vi "Update Application Settings.vi"(6 "wait for reply (T)":bool=TRUE, 8 "error in":errorcluster) -> (0 "error out":errorcluster, 1 "timed out?":bool, 2 "Reply Payload":T1)   [LabVIEW 2020, in "Settings Editor.lvlib"]
doc: "Request Settings Editor to return the latest settings. The Settings Editor can send the applications settings as a reply or via broadcast.\n_____\nCreated using DQMH Event Scripter 4.1.0.75.\n_____\nBased on DQMH Project Template 7.0.1.1316."
uses:
  Settings Editor.lvlib
  Update Application Settings (Reply Payload)--cluster.ctl
  Settings--cluster.ctl
  CML Shared/Signal Type--enum.ctl
  CML Shared/Calibration Values--cluster.ctl
  Update Application Settings Argument--cluster.ctl
  CML Shared/CML Shared.lvlib
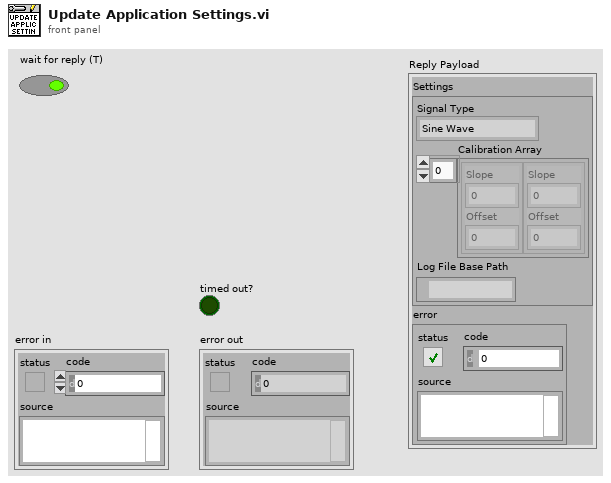
[diagram p1: front panel]
types:
  T1 = typedef "Settings Editor.lvlib/Update Application Settings (Reply Payload)--cluster.ctl" = cluster{"Settings":T2, "error":errorcluster}
  T2 = typedef "Settings Editor.lvlib/Settings--cluster.ctl" = cluster{"Signal Type":T3, "Calibration Array":T4[], "Log File Base Path":path}
  T3 = typedef "CML Shared.lvlib/Signal Type--enum.ctl" = enum16{"Sine Wave", "Square with Noise"}
  T4 = typedef "CML Shared.lvlib/Calibration Values--cluster.ctl" = cluster{"Slope":dbl, "Offset":dbl}
  T5 = typedef "Settings Editor.lvlib/Request Events--cluster.ctl" = cluster{"Stop Module":refnum<user-event>, "Show Panel":refnum<user-event>, "Hide Panel":refnum<user-event>, "Get Module Execution Status":refnum<user-event>, "Show Diagram":refnum<user-event>, "Update Application Settings":refnum<user-event>}
  T6 = typedef "Settings Editor.lvlib/Update Application Settings Argument--cluster.ctl" = cluster{"Wait Notifier":refnum<notifier>, "wait for reply":bool}
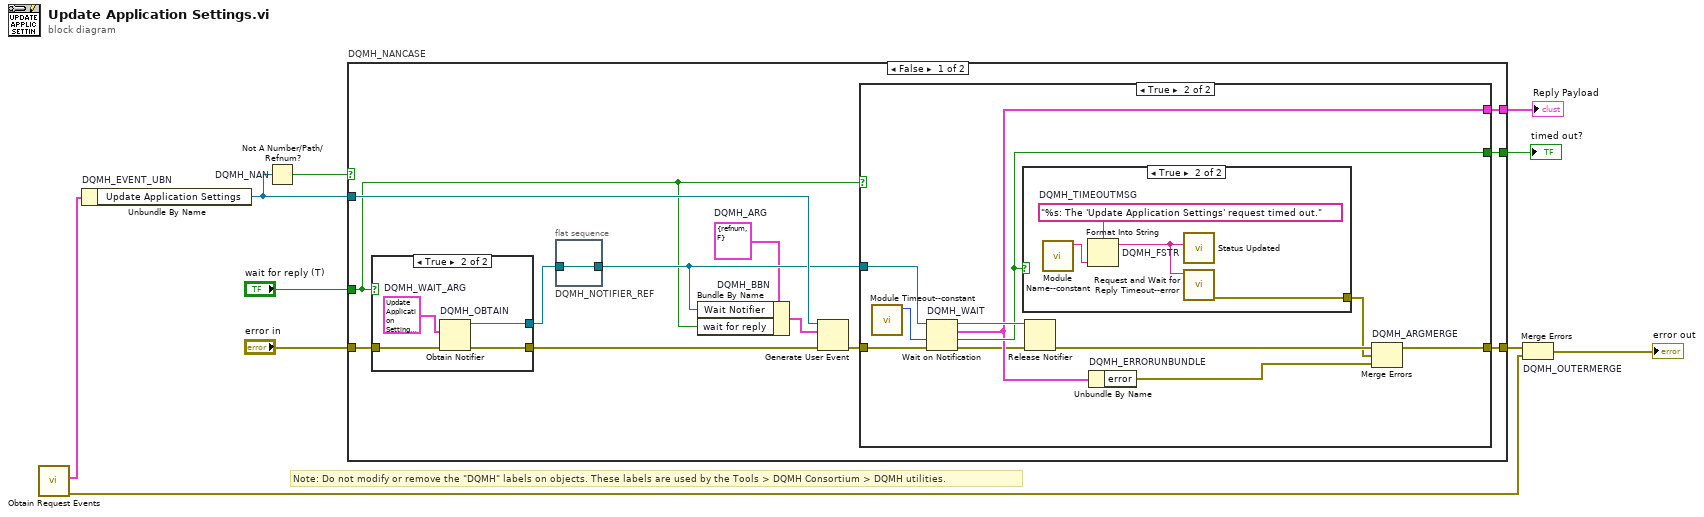
[diagram p0: block diagram]
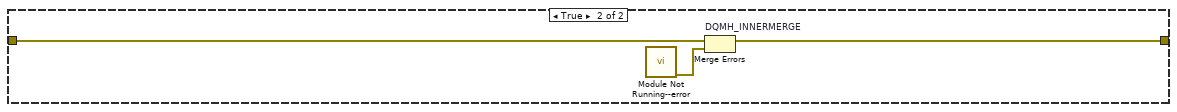
[diagram p5: hidden frame]
diagram:
  # "Note: Do not modify or remove the \"DQMH\" labels on objects. These labels are used by the Tools > DQMH Consortium > DQMH utilities."
  n1 = call "Obtain Request Events.vi"() -> ("error out"=w3:errorcluster, "Settings Editor Request Events"=w2:T5)  [unwired: 10 in]
  n2 = Unbundle By Name "DQMH_EVENT_UBN"(w2) -> ("Update Application Settings"=w8:refnum<user-event>)
  n3 = Not A Number/Path/Refnum? "DQMH_NAN"(number/path/refnum=w8) -> (NaN/Path/Refnum?=w7:bool)
  n4 = case "DQMH_NANCASE" shown="False" w7 {
    tunnel: "error in" -> [w22 w47]
    tunnel: w8 -> [w20 _]
    tunnel: [w17 w46] -> w5
    tunnel: [w18 _] -> w6
    tunnel: "wait for reply (T)" -> [w13 _]
    tunnel: [w11 _] -> w1
    frame False {
      w12 = T6 {"Wait Notifier"=refnum, "wait for reply"=FALSE}  # DQMH_ARG
      n5 = case shown="True" w13 {
        tunnel: w22 -> [w40 w44]
        tunnel: [w40 w43] -> w19
        tunnel: [_ w41] -> w15
        frame False {
        }
        frame True {
          w42 = T1 {"Settings"={"Signal Type"=enum."Sine Wave", "Calibration Array"=[], "Log File Base Path"=path ""}, "error"={"status"=FALSE, "code"=0, "source"=""}}  # DQMH_WAIT_ARG
          n6 = Obtain Notifier "DQMH_OBTAIN"(notification data type=w42, error in (no error)=w44) -> (notifier out=w41:refnum<notifier>, error out=w43:errorcluster)  [unwired: 2 in, 1 out]
        }
      }
      n7 = flat-sequence "DQMH_NOTIFIER_REF" {
        tunnel: w15 -> [w23]
        tunnel: [w23] -> w14
        frame #0 {
        }
      }
      n8 = Bundle By Name "DQMH_BBN"(cluster=w12, "Wait Notifier"=w14, "wait for reply"=w13) -> (w16:T6)
      n9 = Generate User Event(user event=w20, event data cluster=w16, error in=w19) -> (error out=w21:errorcluster)  [unwired: 1 in, 1 out]
      n10 = case shown="True" w13 {
        tunnel: w21 -> [w24 w35]
        tunnel: w14 -> [_ w34]
        tunnel: [_ w32] -> w18
        tunnel: [w24 w31] -> w17
        tunnel: [_ w29] -> w11
        frame False {
        }
        frame True {
          n11 = call "Module Timeout--constant.vi"() -> ("Module Timeout"=w30:i32)  [unwired: 11 in]
          n12 = Wait on Notification "DQMH_WAIT"(notifier=w34, timeout in ms (-1)=w30, error in (no error)=w35) -> (notifier out=w33:refnum<notifier>, notification=w29:T1, timed out?=w32:bool, error out=w28:errorcluster)  [unwired: 1 in]
          n13 = case shown="True" w32 {
            tunnel: [_ w36] -> w25
            frame False {
            }
            frame True {
              w39 = "%s: The 'Update Application Settings' request timed out."  # DQMH_TIMEOUTMSG
              n14 = call "Module Name--constant.vi"() -> ("Module Name"=w38:string)  [unwired: 11 in]
              n15 = Format Into String "DQMH_FSTR"(format string=w39, w38) -> (resulting string=w37:string)  [unwired: 2 in, 1 out]
              n16 = call "Status Updated.vi"("Status"=w37) -> ()  [unwired: 10 in, 1 out]
              n17 = call "Request and Wait for Reply Timeout--error.vi"("Error Message"=w37) -> ("error out"=w36:errorcluster)  [unwired: 10 in]
            }
          }
          n18 = Release Notifier(notifier=w33, error in (no error)=w28) -> (error out=w27:errorcluster)  [unwired: 1 in, 2 out]
          n19 = Unbundle By Name "DQMH_ERRORUNBUNDLE"(w29) -> ("error"=w26:errorcluster)
          n20 = Merge Errors "DQMH_ARGMERGE"(w27, w25, w26) -> (w31:errorcluster)
        }
      }
    }
    frame True {
      n21 = call "Module Not Running--error.vi"() -> ("error out"=w45:errorcluster)  [unwired: 11 in]
      n22 = Merge Errors "DQMH_INNERMERGE"(w47, w45) -> (w46:errorcluster)
    }
  }
  "timed out?" <- w6
  "Reply Payload" <- w1
  n23 = Merge Errors "DQMH_OUTERMERGE"(w5, w3) -> (→"error out":errorcluster)
